vi "save droplet prep info.vi"(6 "Reagent volume (ul)":dbl[](array[numeric]), 7 "Reagent location":dbl[](array[numeric]), 9 "Sample preparation time":string, 10 "Sample name":string, 11 "Exp. file path":path) -> ()   [LabVIEW 2017]
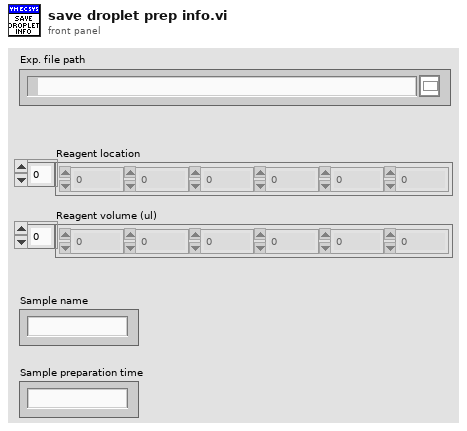
[diagram p1: front panel]
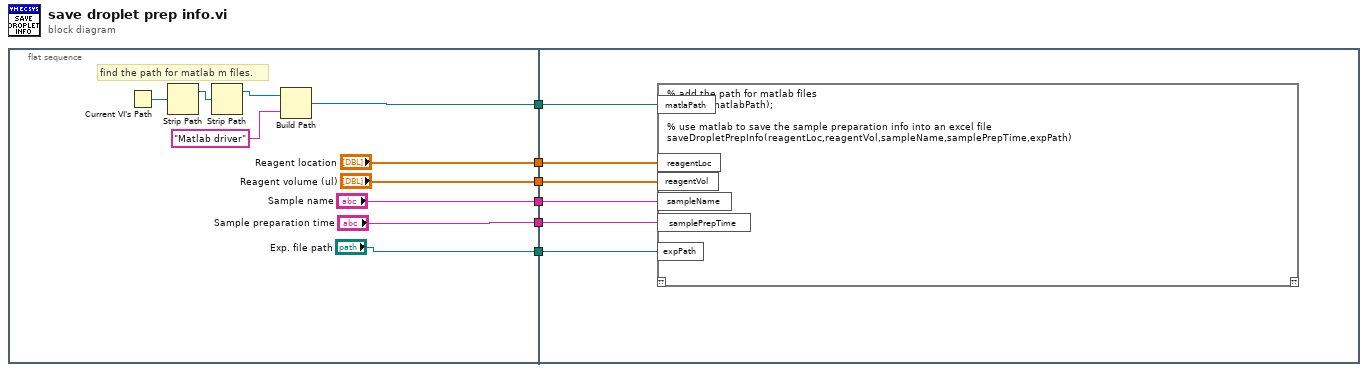
[diagram p0: block diagram]
diagram:
  n1 = flat-sequence {
    tunnel: [w12] -> w6
    tunnel: ["Reagent volume (ul)"] -> w5
    tunnel: ["Reagent location"] -> w4
    tunnel: ["Exp. file path"] -> w3
    tunnel: ["Sample name"] -> w2
    tunnel: ["Sample preparation time"] -> w1
    tunnel: w6 -> [w22]
    tunnel: w5 -> [w21]
    tunnel: w4 -> [w20]
    tunnel: w3 -> [w19]
    tunnel: w2 -> [w18]
    tunnel: w1 -> [w17]
    frame #0 {
      # "find the path for matlab m files."
      n2 = Current VI's Path() -> (path=w16:path)
      n3 = Strip Path(path=w16) -> (stripped path=w15:path)  [unwired: 1 out]
      n4 = Strip Path(path=w15) -> (stripped path=w14:path)  [unwired: 1 out]
      n5 = Build Path(base path=w14, name or relative path="Matlab driver") -> (appended path=w12:path)
    }
    frame #1 {
      n6 = script code="% add the path for matlab files\naddpath(matlabPath);\n\n% use matlab to save the sample preparation info into an excel file\nsaveDropletPrepInfo(reagentLoc,reagentVol,sampleName,samplePrepTime,expPath)"("matlaPath"=w22, "reagentLoc"=w20, "reagentVol"=w21, "sampleName"=w18, "samplePrepTime"=w17, "expPath"=w19) -> ()  [unwired: 1 in, 1 out]
    }
  }
